vi "RP Scale v2.vi"(4 "RP version 2 calibration":bool, 5 "Number of stages":i32=6, 6 "EEPROM offset":i32=78, 7 "Decimation":u32=1, 9 "EEPROM range":u32=45870551, 10 "Signal bits":i32=14, 11 "Range":dbl=1.0 format="%#_6eV") -> (1 "y intersept":dbl, 2 "Calibrated slope":dbl format="%#_27g", 3 "Slope":dbl)   [LabVIEW 2024]
panel:
  out "Calibrated range":dbl
  out "x << y":i32
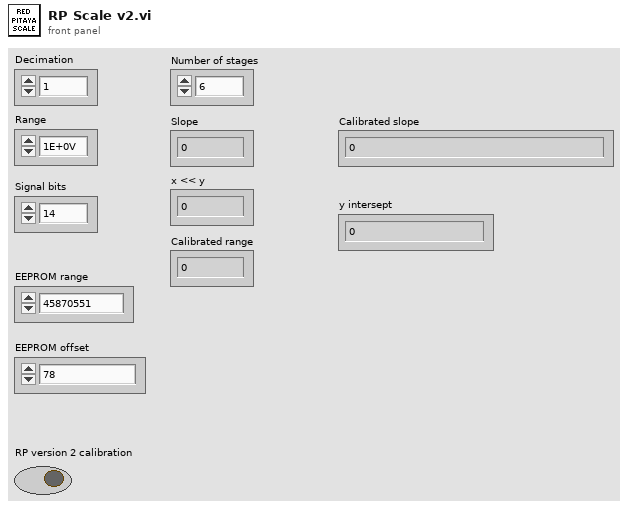
[diagram p1: front panel]
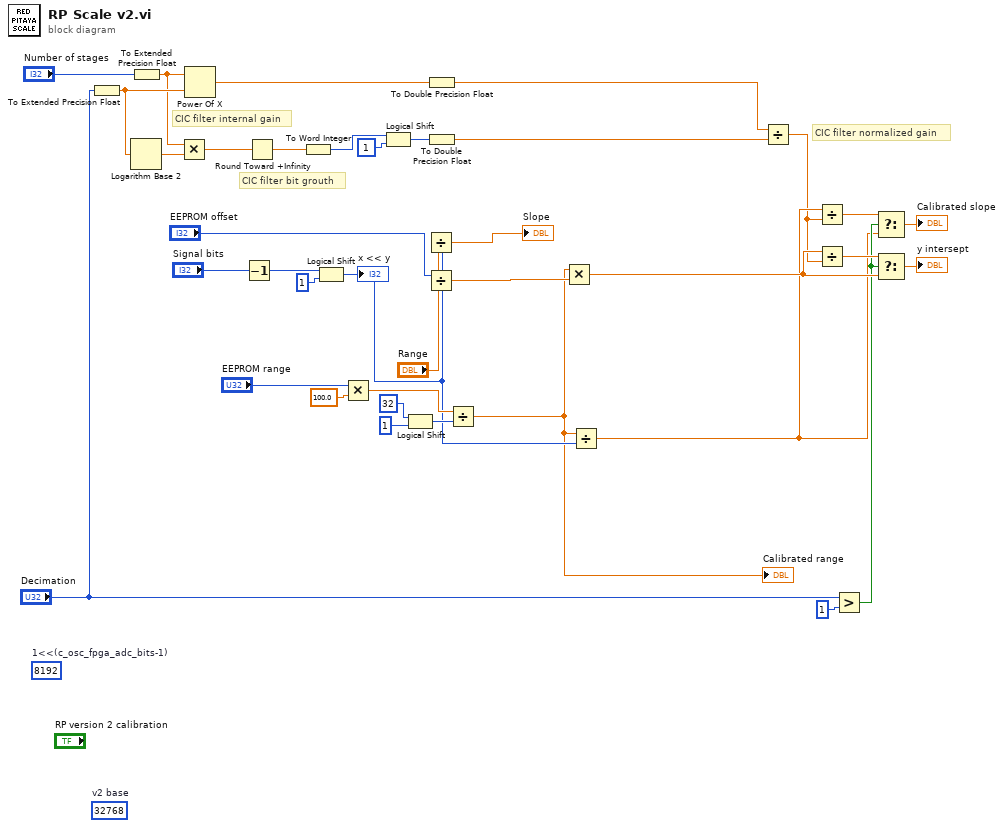
[diagram p0: block diagram]
diagram:
  (unwired) 32768  # v2 base
  (unwired) 8192  # 1<<(c_osc_fpga_adc_bits-1)
  # "CIC filter normalized gain"
  # "CIC filter internal gain"
  # "CIC filter bit grouth"
  n1 = To Extended Precision Float(1:"Decimation") -> (0:w20:ext)
  n2 = Logarithm Base 2(1:w20) -> (0:w18:ext)
  n3 = To Extended Precision Float(1:"Number of stages") -> (0:w19:ext)
  n4 = Multiply(x=w19, y=w18) -> (x*y=w15:ext)
  n5 = Power Of X(1:w20, 2:w19) -> (0:w12:ext)
  n6 = Decrement(x="Signal bits") -> (x-1=w37:i32)
  n7 = Round Toward +Infinity(x=w15) -> (ceil(x): smallest int >= x=w17:ext)
  n8 = To Word Integer(number=w17) -> (16bit integer=w14:i16)
  n9 = Logical Shift(y=w37, x=1) -> (x << y=w23:i32)
  "x << y" <- w23
  n10 = Multiply(x="EEPROM range", y=100.0) -> (x*y=w28:dbl)
  n11 = Logical Shift(y=w14, x=u64 1) -> (x << y=w13:u64)
  n12 = Logical Shift(y=i16 32, x=u64 1) -> (x << y=w27:u64)
  n13 = Divide(x="Range", y=w23) -> (x/y=→"Slope":dbl)
  n14 = Divide(x="EEPROM offset", y=w23) -> (x/y=w25:dbl)
  n15 = To Double Precision Float(number=w12) -> (double precision float=w11:dbl)
  n16 = To Double Precision Float(number=w13) -> (double precision float=w10:dbl)
  n17 = Divide(x=w28, y=w27) -> (x/y=w3:dbl)
  "Calibrated range" <- w3
  n18 = Multiply(x=w3, y=w25) -> (x*y=w24:dbl)
  n19 = Divide(x=w3, y=w23) -> (x/y=w6:dbl)
  n20 = Divide(x=w11, y=w10) -> (x/y=w5:dbl)
  n21 = Divide(x=w6, y=w5) -> (x/y=w8:dbl)
  n22 = Divide(x=w24, y=w5) -> (x/y=w9:dbl)
  n23 = Greater?(x="Decimation", y=u32 1) -> (0:w7:bool)
  n24 = Select(t=w8, s=w7, f=w6) -> (s? t:f=→"Calibrated slope":dbl)
  n25 = Select(t=w9, s=w7, f=w24) -> (s? t:f=→"y intersept":dbl)
